vi "log_template.vi"(4 "接收报文":string="URL=", 6 "a:Success":string, 7 "URL":string="URL=", 8 "StartTime":string, 10 "发送报文":string) -> ()   [LabVIEW 2020]
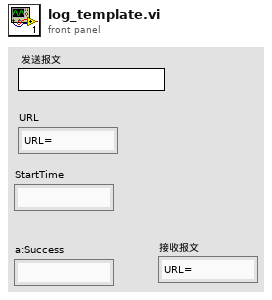
[diagram p1: front panel]
types:
  T1 = enum16{"open", "replace", "create", "open or create", "replace or create", "replace or create with confirmation"}
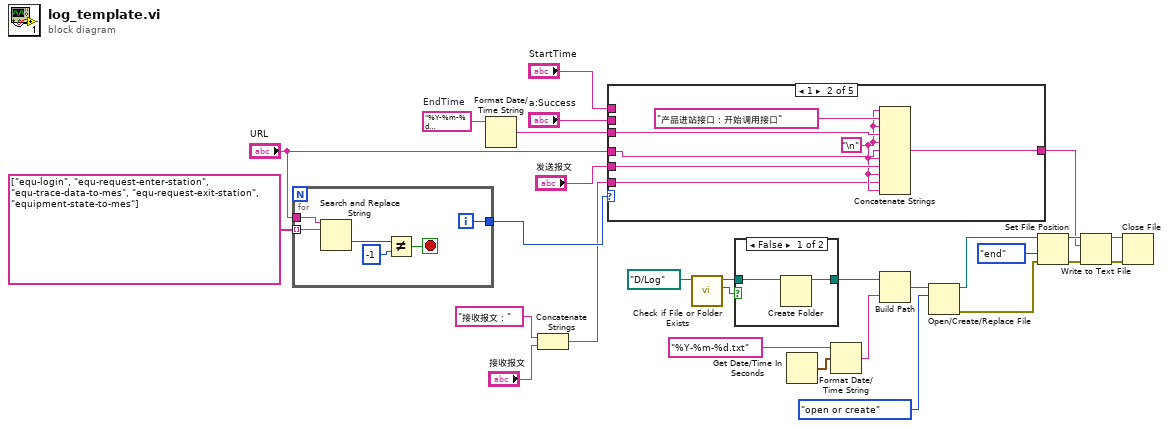
[diagram p0: block diagram]
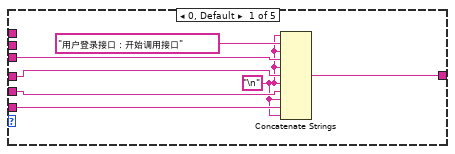
[diagram p2: hidden frame]
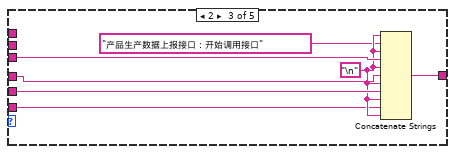
[diagram p3: hidden frame]
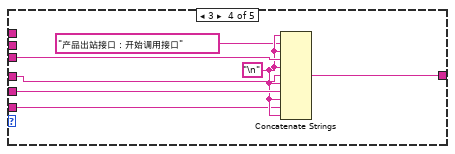
[diagram p4: hidden frame]
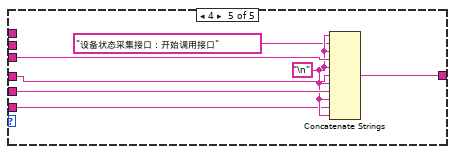
[diagram p5: hidden frame]
diagram:
  w17 = "%Y-%m-%d %H:%M:%S%3u-->"  # EndTime
  n1 = for {
    tunnel: string[] ["equ-login", "equ-request-enter-station", "equ-trace-data-to-mes", "equ-request-exit-station", "equipment-state-to-mes"] ("字符串数组") -> [w30] mode=indexing
    tunnel: "URL" -> [w34]
    tunnel: [w29] -> w20
    i -> [w29]
    stop <- w31 stop-if-true
    n2 = Search and Replace String(input string=w34, search string=w30) -> (offset past replacement=w32:i32)  [unwired: 6 in, 3 out]
    n3 = Not Equal?(x=w32, y=-1) -> (x != y?=w31:bool)
  }
  n4 = Format Date/Time String(time format string (%c)=w17) -> (date/time string=w16:string)  [unwired: 2 in]
  n5 = Concatenate Strings("接收报文：", "接收报文") -> (w1:string)
  n6 = case shown="1" w20 {
    tunnel: "发送报文" -> [w40 w47 w54 w61 w68]
    tunnel: "StartTime" -> [_ _ _ _ _]
    tunnel: w16 -> [w38 w45 w53 w60 w67]
    tunnel: "a:Success" -> [_ _ _ _ _]
    tunnel: w1 -> [w39 w42 w50 w57 w64]
    tunnel: [w41 w48 w55 w62 w69] -> w5
    tunnel: "URL" -> [w37 w43 w51 w58 w65]
    frame 0, Default {
      w35 = "\n"
      n7 = Concatenate Strings(w35, "用户登录接口：开始调用接口", w35, w38, w35, w37, w35, w40, w35, w39, w35) -> (w41:string)
    }
    frame 1 {
      w44 = "\n"
      n8 = Concatenate Strings(w44, "产品进站接口：开始调用接口", w44, w45, w44, w43, w44, w47, w44, w42, w44) -> (w48:string)
    }
    frame 2 {
      w52 = "\n"
      n9 = Concatenate Strings(w52, "产品生产数据上报接口：开始调用接口", w52, w53, w52, w51, w52, w54, w52, w50, w52) -> (w55:string)
    }
    frame 3 {
      w59 = "\n"
      n10 = Concatenate Strings(w59, "产品出站接口：开始调用接口", w59, w60, w59, w58, w59, w61, w59, w57, w59) -> (w62:string)
    }
    frame 4 {
      w66 = "\n"
      n11 = Concatenate Strings(w66, "设备状态采集接口：开始调用接口", w66, w67, w66, w65, w66, w68, w66, w64, w66) -> (w69:string)
    }
  }
  n12 = call <vilib>:"Check if File or Folder Exists.vi"("path"=path "D:/Log" ("路径")) -> ("file or folder exists?"=w26:bool, "dup path"=w27:path)  [unwired: 8 in, 1 out]
  n13 = case shown="False" w26 {
    tunnel: w27 -> [w71 w72]
    tunnel: [w70 w72] -> w24
    frame False {
      n14 = Create Folder(path (use dialog)=w71) -> (created path=w70:path)  [unwired: 2 in, 2 out]
    }
    frame True {
    }
  }
  n15 = Get Date/Time In Seconds() -> (seconds since 1Jan1904=w22:timestamp)
  n16 = Format Date/Time String(time format string (%c)="%Y-%m-%d.txt" ("时间格式字符串(%c)"), seconds (now)=w22) -> (date/time string=w21:string)  [unwired: 1 in]
  n17 = Build Path(base path=w24, name or relative path=w21) -> (appended path=w28:path)
  n18 = Open/Create/Replace File(file path (use dialog)=w28, operation (0:open)=T1."open or create" ("操作(0:open)")) -> (refnum out=w10:refnum<file>, error out=w11:errorcluster)  [unwired: 4 in, 1 out]
  n19 = Set File Position(refnum=w10, from (0:start)=enum16{"start", "end", "current"}."end" ("自（0:起始）"), error in=w11) -> (refnum out=w12:refnum<file>, error out=w13:errorcluster)  [unwired: 1 in]
  n20 = Write to Text File(file (use dialog)=w12, text=w5, error in=w13) -> (refnum out=w9:refnum<file>, error out=w8:errorcluster)  [unwired: 1 in, 1 out]
  n21 = Close File(refnum=w9, error in=w8) -> ()  [unwired: 2 out]
